vi "Array to Multi Ch XYPlots.vi"(8 "channel names":string[](array[string]), 10 "Y array":dbl[](array[numeric]), 11 "X array":dbl[](array[numeric])) -> (3 "XY plots":cluster{"X array":dbl[], "Y array":dbl[]}[](array[cluster]))   [LabVIEW 2021]
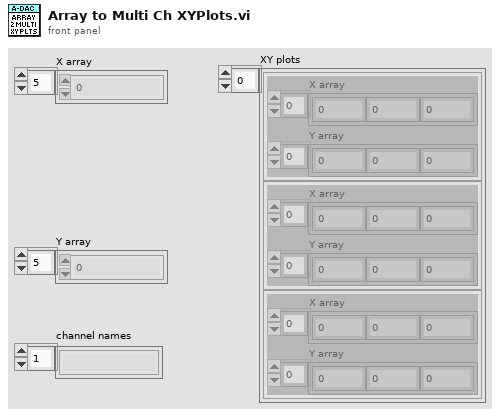
[diagram p1: front panel]
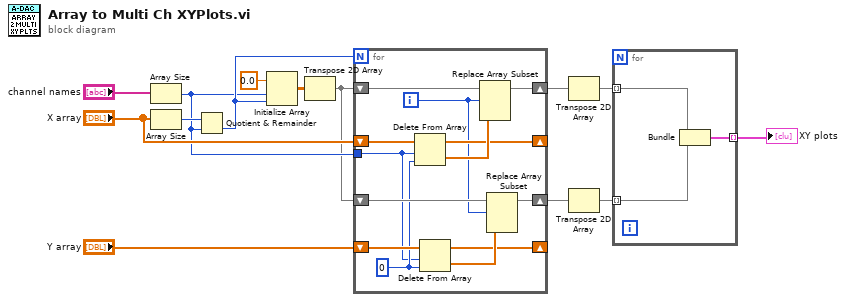
[diagram p0: block diagram]
diagram:
  n1 = Array Size(array="channel names") -> (size(s)=w8:i32)
  n2 = Array Size(array="X array") -> (size(s)=w11:i32)
  n3 = Quotient & Remainder(x=w11, y=w8) -> (floor(x/y)=w9:i32)  [unwired: 1 out]
  n4 = Initialize Array(0.0 ("element"), w8, w9) -> (w12:dbl[][])
  n5 = Transpose 2D Array(2D array=w12) -> (transposed array=w7:dbl[][])
  n6 = for {
    N: w9 -> [_]
    shift-right: [w26] -> w5
    shift-left: w7 -> [w27]
    tunnel: w8 -> [w17]
    shift-right: [w23] -> _
    shift-left: "X array" -> [w25]
    shift-right: [w21] -> w4
    shift-left: w7 -> [w22]
    shift-right: [w15] -> _
    shift-left: "Y array" -> [w19]
    i -> [w20]
    w18 = 0 ("index")
    n7 = Delete From Array(array=w25, length=w17, index=w18) -> (deleted portion=w24:dbl[], array with subset deleted=w23:dbl[])
    n8 = Delete From Array(array=w19, length=w17, index=w18) -> (deleted portion=w16:dbl[], array with subset deleted=w15:dbl[])
    n9 = Replace Array Subset(array=w27, new element=w24, index (row)=w20) -> (w26:dbl[][])  [unwired: 1 in]
    n10 = Replace Array Subset(array=w22, new element=w16, index (row)=w20) -> (w21:dbl[][])  [unwired: 1 in]
  }
  n11 = Transpose 2D Array(2D array=w5) -> (transposed array=w3:dbl[][])
  n12 = Transpose 2D Array(2D array=w4) -> (transposed array=w2:dbl[][])
  n13 = for {
    tunnel: w3 -> [w30] mode=indexing
    tunnel: w2 -> [w29] mode=indexing
    tunnel: [w28] -> w1 mode=indexing
    n14 = Bundle(w30, w29) -> (w28:cluster{dbl[], dbl[]})  [unwired: 1 in]
  }
  "XY plots" <- w1
